vi "Serrure numérique.vi"() -> ()   [LabVIEW 2018]
panel:
  out "Boolean":bool
  in  "Knob 3":i8(knob) scale=0.0..10.0
  in  "Knob 2":i8(knob) scale=0.0..10.0
  in  "Knob":i8(knob) scale=0.0..10.0
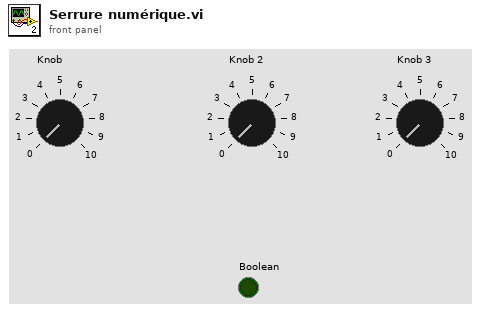
[diagram p1: front panel]
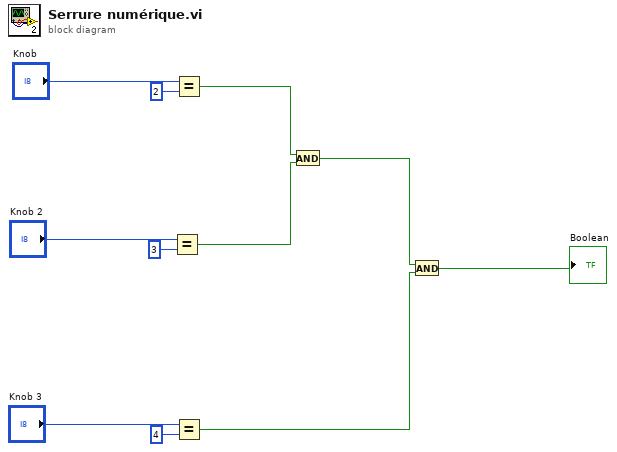
[diagram p0: block diagram]
diagram:
  n1 = Equal?(x="Knob 2", y=i8 3) -> (x = y?=w4:bool)
  n2 = Equal?(x="Knob", y=i8 2) -> (x = y?=w5:bool)
  n3 = Equal?(x="Knob 3", y=i8 4) -> (x = y?=w2:bool)
  n4 = And(x=w5, y=w4) -> (x .and. y?=w3:bool)
  n5 = And(x=w3, y=w2) -> (x .and. y?=→"Boolean":bool)
